vi "Component Thickness.vi"() -> ()   [LabVIEW 2018]
panel:
  in  "Numeric":dbl
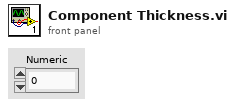
[diagram p1: front panel]
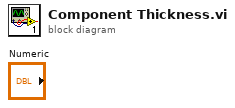
[diagram p0: block diagram]
diagram:
